vi "Get Property List.vi"(8 "error in (no error)":errorcluster caption="错误输入（无错误）", 11 "Item输入":refnum<class "Item.lvclass">) -> (0 "error out":errorcluster caption="错误输出", 1 "Values":variant[](array[variant]), 2 "Property Names":string[](array[string]), 3 "Item输出":refnum<class "Item.lvclass">)   [LabVIEW 2013, in "Hierarchy Framework.lvlib" / "Item.lvclass"]
doc: "Returns all the <B>Property Names</B> and <B>Values</B> of the properties associated with a custom device item."
uses:
  Item.lvclass
  Item.lvclass/Item.ctl
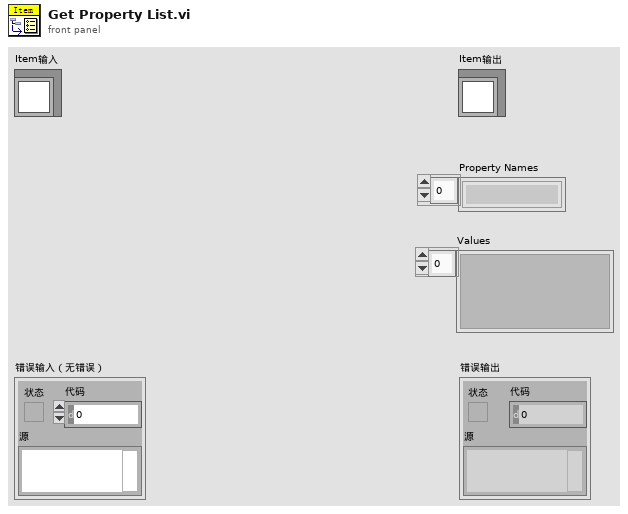
[diagram p1: front panel]
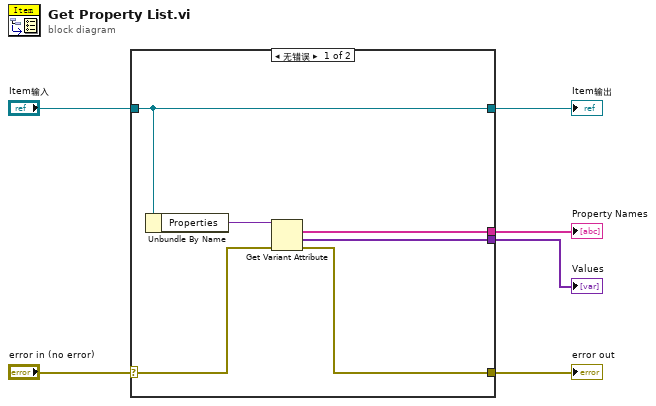
[diagram p0: block diagram]
diagram:
  n1 = case shown="无错误" "error in (no error)" {
    selector: "error in (no error)" -> [w9 w14]
    tunnel: [w8 w14] -> w5
    tunnel: [w12 w13] -> w3
    tunnel: "Item输入" -> [w12 w13]
    tunnel: [w10 _] -> w2
    tunnel: [w7 _] -> w1
    frame No Error {
      n2 = Unbundle By Name(w12) -> ("Properties"=w11:variant)
      n3 = Get Variant Attribute(Variant=w11, error in=w9) -> (names=w10:string[], values=w7:variant[], error out=w8:errorcluster)  [unwired: 2 in, 1 out]
    }
    frame Error {
    }
  }
  "error out" <- w5
  "Item输出" <- w3
  "Property Names" <- w2
  "Values" <- w1
